vi "Initialize.vi"(8 "error in (no error)":errorcluster, 9 "Reset (F)":bool, 10 "IdQuery (F)":bool, 11 "NiPxi6733 in":refnum<class "NiPxi6733.lvclass">) -> (0 "error out":errorcluster, 3 "NiPxi6733 out":refnum<class "NiPxi6733.lvclass">)   [LabVIEW 2014, in "FgenPlugins.lvlib" / "NiPxi6733.lvclass"]
uses:
  NiPxi6733.lvclass
  FgenPluginBaseClass/FgenPluginsBase.lvclass/FgenPluginsBase.ctl
  FgenPluginBaseClass/Accessors/Read Channels.vi
  FgenPluginBaseClass/Accessors/Write Channels.vi
  <vilib>/DAQmx/create/channels.llb/DAQmx Create Channel (AO-Voltage-Basic).vi
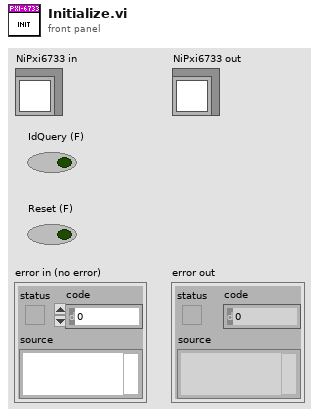
[diagram p1: front panel]
types:
  T1 = cluster{bool, "instrument handle out":refnum<k21>}[]
  T2 = typedef "FgenPlugins.lvlib/Channel.ctl" = cluster{"Name":string, "Enabled":bool, "Operation":enum16{"Continuous", "Burst"}, "Impedance (50)":dbl, "Handle":string, "Connected":bool, "Mode (Function)":enum16{"Function", "Arbitrary", "Sequence"}}
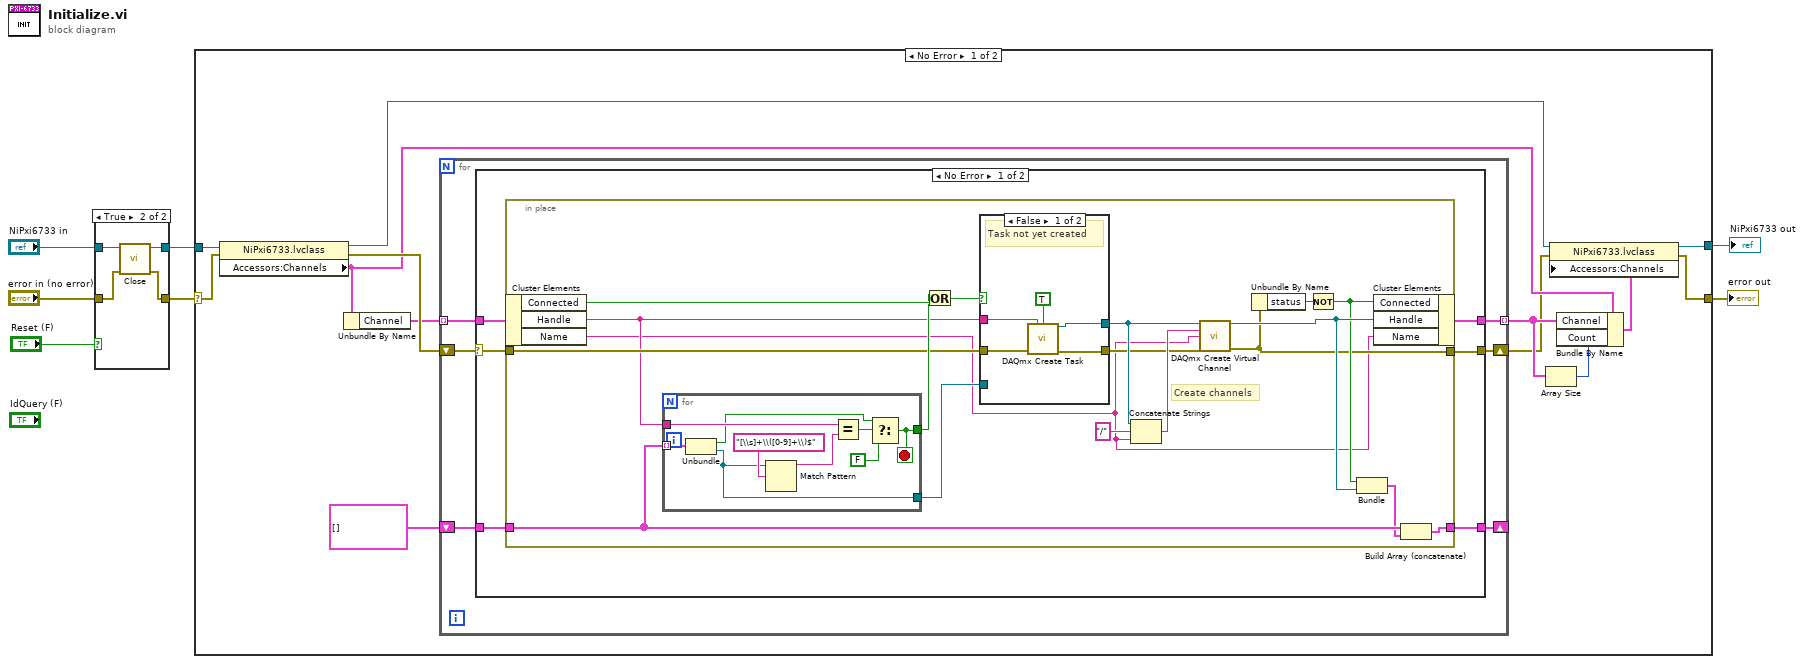
[diagram p0: block diagram]
diagram:
  n1 = case shown="True" "Reset (F)" {
    tunnel: [w9 w13] -> w5
    tunnel: "NiPxi6733 in" -> [w9 w12]
    tunnel: "error in (no error)" -> [w8 w11]
    tunnel: [w8 w10] -> w2
    frame False {
    }
    frame True {
      n2 = call-dynamic "Close.vi"("error in (no error)"=w11, "NiPxi6733 in"=w12) -> ("error out"=w10:errorcluster, "NiPxi6733 out"=w13:refnum<class "NiPxi6733.lvclass">)  [unwired: 8 in]
    }
  }
  n3 = case shown="No Error" w2 {
    selector: w2 -> [w25 w76]
    tunnel: [w15 w77] -> w7
    tunnel: w5 -> [w26 w77]
    tunnel: [w14 w76] -> w6
    frame No Error {
      n4 = property class="NiPxi6733.lvclass"(reference=w26, error in=w25) -> (reference out=w16:refnum<class "NiPxi6733.lvclass">, error out=w24:errorcluster, "Accessors:Channels"=w21:cluster{"Count":u16, "Channel":T2[]})
      n5 = Unbundle By Name(w21) -> ("Channel"=w22:T2[])
      n6 = for {
        tunnel: w22 -> [w32] mode=indexing
        shift-right: [w28] -> w17
        shift-left: w24 -> [w30]
        shift-right: [w29] -> _
        shift-left: T1 [] -> [w31]
        tunnel: [w27] -> w18 mode=indexing
        n7 = case shown="No Error" w30 {
          selector: w30 -> [w36 w75]
          tunnel: w32 -> [w38 w73]
          tunnel: w31 -> [w37 w74]
          tunnel: [w35 w74] -> w29
          tunnel: [w34 w75] -> w28
          tunnel: [w33 w73] -> w27
          frame No Error {
            n8 = in-place {
              in-place-border: w37 -> [w52]
              in-place-border: w36 -> [w53]
              in-place-border: [w49] -> w35
              in-place-border: [w40] -> w34
              # "Create channels"
              n9 = in-place-cluster #1(w38) -> ("Connected"=w56:bool, "Handle"=w48:string, "Name"=w39:string)
              n10 = for {
                tunnel: w48 -> [w70]
                tunnel: w52 -> [w72] mode=indexing
                tunnel: [w65] -> w55
                tunnel: [w64] -> w51
                stop <- w65 stop-if-true
                n11 = Unbundle(w72) -> (w66:bool, "instrument handle out"=w64:refnum<k21>)
                n12 = Match Pattern(string=w64, regular expression="[\\s]+\\([0-9]+\\)$") -> (before substring=w69:string)  [unwired: 1 in, 3 out]
                n13 = Equal?(x=w70, y=w69) -> (x = y?=w68:bool)
                n14 = Select(t=w66, s=w68, f=FALSE) -> (s? t:f=w65:bool)
              }
              n15 = Or(x=w55, y=w56) -> (x .or. y?=w54:bool)
              n16 = case shown="False" w54 {
                tunnel: w53 -> [w60 w63]
                tunnel: [w58 w63] -> w43
                tunnel: w51 -> [_ w62]
                tunnel: [w57 w62] -> w44
                tunnel: w48 -> [w59 _]
                frame False {
                  # "Task not yet created"
                  n17 = call <vilib>:"DAQmx Create Task.vi"("new task name"=w59, "auto cleanup"=TRUE, "error in"=w60) -> ("task out"=w57:refnum<k21>, "error out"=w58:errorcluster)  [unwired: 11 in]
                }
                frame True {
                  # "Task has been created"
                }
              }
              n18 = Concatenate Strings(w44, "/" ("string"), w39) -> (w45:string)
              n19 = call-poly <vilib>:"DAQmx Create Virtual Channel.vi"("task in"=w44, "physical channels"=w45, "name to assign"=w39, "error in"=w43) -> ("task out"=w42:refnum<k21>, "error out"=w40:errorcluster)  [unwired: 10 in]
              n20 = Unbundle By Name(w40) -> ("status"=w47:bool)
              n21 = Not(x=w47) -> (.not. x?=w41:bool)
              n22 = Bundle(w41, "task out"=w42) -> (w50:cluster{bool, "task out":refnum<k21>})  [unwired: 1 in]
              n23 = in-place-cluster #1("Connected"=w41, "Handle"=w42, "Name"=w39) -> (w33:T2)
              n24 = Build Array (concatenate)(w52, w50) -> (w49:cluster{bool, "task out":refnum<k21>}[])
            }
          }
          frame Error {
          }
        }
      }
      n25 = Array Size(array=w18) -> (size(s)=w19:i32)
      n26 = Bundle By Name(cluster=w21, "Channel"=w18, "Count"=w19) -> (w20:cluster{"Count":u16, "Channel":T2[]})
      n27 = property class="NiPxi6733.lvclass"(reference=w16, error in=w17, "Accessors:Channels"=w20) -> (reference out=w15:refnum<class "NiPxi6733.lvclass">, error out=w14:errorcluster)
    }
    frame Error {
    }
  }
  "error out" <- w6
  "NiPxi6733 out" <- w7
